vi "PathPlanner_ReadTrajectory_CSV_FIle_Global_Example.vi"() -> ()   [LabVIEW 2019]
uses:
  SubVI/pathplanner_read_csv_GlobalVariable.vi
panel:
  out "error out":errorcluster
  # "Read Trajectory CSV File and \nWrite to Global Variable"
  # "See block diagram"
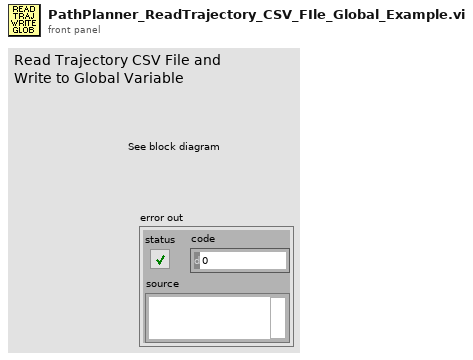
[diagram p1: front panel]
types:
  T1 = typedef "PathPlanner24.lvlib/PathPlannerTrajectory.ctl" = cluster{"States":T2[]}
  T2 = typedef "PathPlanner24.lvlib/PathPlannerTrajectoryState.ctl" = cluster{"TimeSeconds":dbl, "VelocityMPS":dbl, "AccerationMpsSq":dbl, "HeadingAngularVelRadPerSec":dbl, "PositionMeters":T3, "Heading":T4, "TargetHolonomicRotation":T4, "CurvatureRadPerMeter":dbl, "PathPlannerConstraints":T5, "DeltaPos":dbl}
  T3 = typedef "Trajectory_Library.lvlib/TRANSLATION2D.ctl" = cluster{"X":dbl, "Y":dbl}
  T4 = typedef "Trajectory_Library.lvlib/ROTATION2D.ctl" = cluster{"VALUE":dbl, "COS":dbl, "SIN":dbl}
  T5 = typedef "PathPlanner24.lvlib/PathPlannerPathConstraints.ctl" = cluster{"MaxVelocityMps;":dbl, "MaxAccelerationMpsSq;":dbl, "MaxAngularVelRadPsEc;":dbl, "MaxAngularAccRadPSecSq":dbl, "Exists":bool}
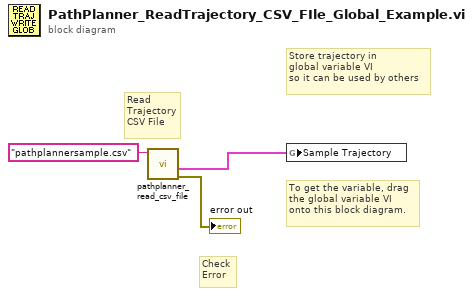
[diagram p0: block diagram]
diagram:
  # "Check\nError"
  # "Read\nTrajectory\nCSV File"
  # "To get the variable, drag\nthe global variable VI\nonto this block diagram."
  # "Store trajectory in\nglobal variable VI\nso it can be used by others"
  n1 = call "pathplanner_read_csv_file.vi"("CSV File Name"="pathplannersample.csv") -> ("error out"=→"error out":errorcluster, "Path Planner Trajectory"=w1:T1)  [unwired: 7 in, 2 out]
  n2 = global write "pathplanner_read_csv_GlobalVariable.vi" "Sample Trajectory"(w1) -> ()
